vi "ShoulderGetSetpointValue.vi"(8 "SholdrSetpoints":T1=enum."ArmFloorPickup") -> (0 "Setpoint":dbl)   [LabVIEW 2023]
doc: "Gets arm position depending enum value"
uses:
  ShoulderGetSetpointEnum.ctl
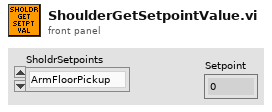
[diagram p1: front panel]
types:
  T1 = typedef "ShoulderGetSetpointEnum.ctl" = enum16{"ShoulderRest", "ShoulderShoot", "ShoulderAmp", "ArmFloorPickup", "ArmAmpDeposit", "ArmSpeakerShoot", "ArmStartPosition", "ArmRestPosition", "ArmSourceIntake", "ArmAwayShoot"}
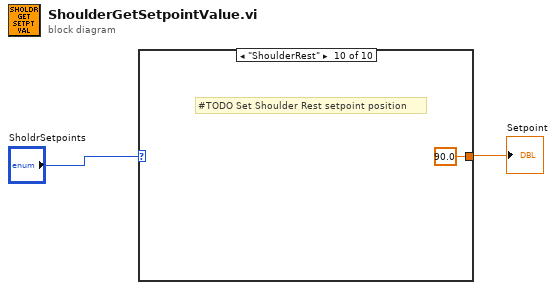
[diagram p0: block diagram]
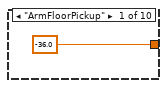
[diagram p2: hidden frame]
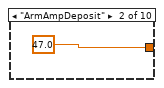
[diagram p3: hidden frame]
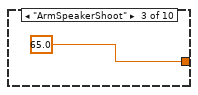
[diagram p4: hidden frame]
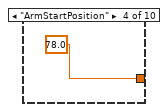
[diagram p5: hidden frame]
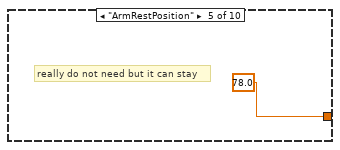
[diagram p6: hidden frame]
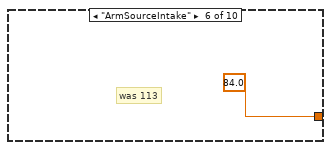
[diagram p7: hidden frame]
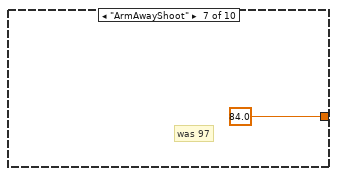
[diagram p8: hidden frame]
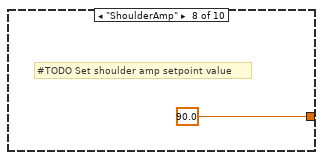
[diagram p9: hidden frame]
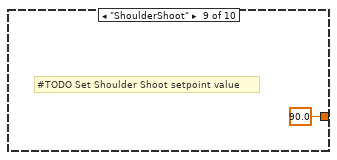
[diagram p10: hidden frame]
diagram:
  n1 = case shown="\"ShoulderRest\"" "SholdrSetpoints" {
    tunnel: [-36.0 ("y") 47.0 ("y") 65.0 ("y") 78.0 ("y") 78.0 ("y") 84.0 ("y") 84.0 ("y") 90.0 ("y") 90.0 ("y") 90.0 ("y")] -> w1
    frame "ArmFloorPickup" {
    }
    frame "ArmAmpDeposit" {
    }
    frame "ArmSpeakerShoot" {
    }
    frame "ArmStartPosition" {
    }
    frame "ArmRestPosition" {
      # "really do not need but it can stay"
    }
    frame "ArmSourceIntake" {
      # "was 113"
    }
    frame "ArmAwayShoot" {
      # "was 97"
    }
    frame "ShoulderAmp" {
      # "#TODO Set shoulder amp setpoint value"
    }
    frame "ShoulderShoot" {
      # "#TODO Set Shoulder Shoot setpoint value"
    }
    frame "ShoulderRest" {
      # "#TODO Set Shoulder Rest setpoint position"
    }
  }
  "Setpoint" <- w1
